vi "Process.vi"(8 "error in":errorcluster, 11 "Example Instrument UI":refnum<class "Instrument UI.LN2.lvclass">) -> (0 "error out":errorcluster, 3 "Example Instrument UI out":refnum<class "Instrument UI.LN2.lvclass">)   [LabVIEW 2019, in "Instrument UI.LN2.lvclass"]
doc: "---------------------------------------------------------------\nJKI State Machine Objects™\nhttp://jki.net/state-machine-objects/\nCopyright (C) 2005-2015, JKI <info@jki.net>\nALL RIGHTS RESERVEDJKI State Machine Objects (SMO) 1.0.0.5\nJKI - JKI\nCopyright (c) 2016, JKI"
uses:
  Instrument UI.LN2.lvclass
  C:/Program Files (x86)/National Instruments/LabVIEW 2019/vi.lib/JKI/JKI SMO/SMO/SMO.lvclass
  C:/Program Files (x86)/National Instruments/LabVIEW 2019/user.lib/LevyLab/Instrument Framework/SMOs/Instrument UI/Instrument UI.lvclass
  C:/Program Files (x86)/National Instruments/LabVIEW 2019/vi.lib/JKI/JKI SMO/SMO.UI/SMO.UI.lvclass
  Instrument.LN2/Typedefs/Instrument.LN2.getAll--Cluster.ctl
  Instrument.LN2/Instrument.LN2.lvclass
  C:/Program Files (x86)/National Instruments/LabVIEW 2019/user.lib/LevyLab/Instrument Framework/SMOs/Instrument/Instrument.lvclass
  Instrument UI.LN2.UI--Cluster.ctl
  Instrument.LN2/Typedefs/Instrument.LN2.Configuration--Cluster.ctl
  <userlib>/LevyLab/Instrument Framework/SMOs/Configuration/Configuration.lvclass
  <userlib>/LevyLab/Instrument Framework/SMOs/Instrument UI/Instrument UI.lvclass/Instrument UI.ctl
  <vilib>/JKI/JKI SMO/SMO/SMO.lvclass/SMO.ctl
  <userlib>/LevyLab/Instrument Framework/SMOs/Configuration/Configuration.lvclass/Configuration.ctl
  <userlib>/LevyLab/Instrument Framework/SMOs/Instrument/Instrument.lvclass/Instrument.ctl
  570207f0-e501-44f0-9618-964b5be4b2e0.vi
  064e3a37-d4cf-416d-9c97-81a00de9d50c.vi
  3ac88aea-1a9b-4987-becd-cafda593f7dd.vi
  <vilib>/JKI/JKI SMO/SMO/Private/ReftoDVR--SMO.vi
  570207f0-e501-44f0-9618-964b5be4b2e0.vi/caf046b2-5564-4fc5-9988-a6deaa861af8.vi
  064e3a37-d4cf-416d-9c97-81a00de9d50c.vi/e94c7b98-807a-4028-bf59-40b0245fb82b.vi
  3ac88aea-1a9b-4987-becd-cafda593f7dd.vi/dcf467b4-f1e1-4b46-b912-9ef69395c1ef.vi
  <userlib>/LevyLab/Instrument Framework/SMOs/Instrument/API/Send and Receive.vi
  3ac88aea-1a9b-4987-becd-cafda593f7dd.vi/87cdbc2a-7ef5-4e78-ae8f-77a685c984f9.vi
  <userlib>/LevyLab/Instrument Framework/SMOs/Instrument/Private/Get Client Type.vi
  570207f0-e501-44f0-9618-964b5be4b2e0.vi/caf046b2-5564-4fc5-9988-a6deaa861af8.vi/24e8312f-bad0-4d20-b7ce-0262f896184e.vi
  570207f0-e501-44f0-9618-964b5be4b2e0.vi/caf046b2-5564-4fc5-9988-a6deaa861af8.vi/d2585e3b-91c6-4f37-8627-ecef36f0e358.vi
  064e3a37-d4cf-416d-9c97-81a00de9d50c.vi/e94c7b98-807a-4028-bf59-40b0245fb82b.vi/ea1ec72b-e595-4509-9838-8d04b7e19cf0.vi
  064e3a37-d4cf-416d-9c97-81a00de9d50c.vi/e94c7b98-807a-4028-bf59-40b0245fb82b.vi/ca603f86-ca35-4c9c-a60a-82e1144c324f.vi
  3ac88aea-1a9b-4987-becd-cafda593f7dd.vi/dcf467b4-f1e1-4b46-b912-9ef69395c1ef.vi/e6b65ff1-2ffe-43b7-9398-b93f85180f35.vi
  3ac88aea-1a9b-4987-becd-cafda593f7dd.vi/dcf467b4-f1e1-4b46-b912-9ef69395c1ef.vi/e65e6366-964f-4408-b43e-2679365e4603.vi
  3ac88aea-1a9b-4987-becd-cafda593f7dd.vi/87cdbc2a-7ef5-4e78-ae8f-77a685c984f9.vi/814d43a9-fe47-4414-b08c-5bce024554fc.vi
  3ac88aea-1a9b-4987-becd-cafda593f7dd.vi/87cdbc2a-7ef5-4e78-ae8f-77a685c984f9.vi/5fb6644c-4c1d-4bef-b719-91b55b7f173d.vi
  570207f0-e501-44f0-9618-964b5be4b2e0.vi/caf046b2-5564-4fc5-9988-a6deaa861af8.vi/24e8312f-bad0-4d20-b7ce-0262f896184e.vi/2d73064b-1846-4431-93a5-eb87277d2863.vi
  570207f0-e501-44f0-9618-964b5be4b2e0.vi/caf046b2-5564-4fc5-9988-a6deaa861af8.vi/24e8312f-bad0-4d20-b7ce-0262f896184e.vi/96192298-3fd9-4fdc-9165-8347bdbd3bd8.vi
  570207f0-e501-44f0-9618-964b5be4b2e0.vi/caf046b2-5564-4fc5-9988-a6deaa861af8.vi/d2585e3b-91c6-4f37-8627-ecef36f0e358.vi/2d53ec29-cb0a-4d87-bfb8-ac7d7758049e.vi
  570207f0-e501-44f0-9618-964b5be4b2e0.vi/caf046b2-5564-4fc5-9988-a6deaa861af8.vi/d2585e3b-91c6-4f37-8627-ecef36f0e358.vi/68b74ad3-6d49-41d6-a3f9-22d3dbfe5c7c.vi
  064e3a37-d4cf-416d-9c97-81a00de9d50c.vi/e94c7b98-807a-4028-bf59-40b0245fb82b.vi/ea1ec72b-e595-4509-9838-8d04b7e19cf0.vi/e084a756-656f-4cb3-b7ce-ba8ae6e9a3ed.vi
  064e3a37-d4cf-416d-9c97-81a00de9d50c.vi/e94c7b98-807a-4028-bf59-40b0245fb82b.vi/ea1ec72b-e595-4509-9838-8d04b7e19cf0.vi/8cc34da9-8e4d-45ae-b786-ca14aa9f429e.vi
  064e3a37-d4cf-416d-9c97-81a00de9d50c.vi/e94c7b98-807a-4028-bf59-40b0245fb82b.vi/ca603f86-ca35-4c9c-a60a-82e1144c324f.vi/edcbe473-f127-4b1e-aea6-5a49f1961ddd.vi
  064e3a37-d4cf-416d-9c97-81a00de9d50c.vi/e94c7b98-807a-4028-bf59-40b0245fb82b.vi/ca603f86-ca35-4c9c-a60a-82e1144c324f.vi/9a19d119-1846-4deb-b3ac-a3b5d50ecf35.vi
  3ac88aea-1a9b-4987-becd-cafda593f7dd.vi/87cdbc2a-7ef5-4e78-ae8f-77a685c984f9.vi/814d43a9-fe47-4414-b08c-5bce024554fc.vi/aa77fdb9-b955-481b-814e-f9653af26bf2.vi
  3ac88aea-1a9b-4987-becd-cafda593f7dd.vi/87cdbc2a-7ef5-4e78-ae8f-77a685c984f9.vi/814d43a9-fe47-4414-b08c-5bce024554fc.vi/eac67a51-df62-4b9b-b6ca-6b8735c11697.vi
  570207f0-e501-44f0-9618-964b5be4b2e0.vi/caf046b2-5564-4fc5-9988-a6deaa861af8.vi/d2585e3b-91c6-4f37-8627-ecef36f0e358.vi/2d53ec29-cb0a-4d87-bfb8-ac7d7758049e.vi/17da7eab-c41b-4105-b235-6a3dd260d5b4.vi
  570207f0-e501-44f0-9618-964b5be4b2e0.vi/caf046b2-5564-4fc5-9988-a6deaa861af8.vi/d2585e3b-91c6-4f37-8627-ecef36f0e358.vi/2d53ec29-cb0a-4d87-bfb8-ac7d7758049e.vi/4a0639b9-f07b-4c56-94f4-68eb7f7105d7.vi
  064e3a37-d4cf-416d-9c97-81a00de9d50c.vi/e94c7b98-807a-4028-bf59-40b0245fb82b.vi/ca603f86-ca35-4c9c-a60a-82e1144c324f.vi/edcbe473-f127-4b1e-aea6-5a49f1961ddd.vi/a9985013-86db-4bf4-88b6-4de333bcf681.vi
  064e3a37-d4cf-416d-9c97-81a00de9d50c.vi/e94c7b98-807a-4028-bf59-40b0245fb82b.vi/ca603f86-ca35-4c9c-a60a-82e1144c324f.vi/edcbe473-f127-4b1e-aea6-5a49f1961ddd.vi/f3a922f7-f720-4162-b0c1-e020b75b8308.vi
  <userlib>/LevyLab/Instrument Framework/SMOs/Instrument/Private/Get RC Connection Status.vi
  <userlib>/LevyLab/Instrument Framework/SMOs/Instrument/API/Enum to String.vi
  <userlib>/LevyLab/Instrument Framework/SMOs/RemoteControl/API/Send and Receive.vi
  <vilib>/Utility/Data Type/Get Type Information.vi
  <vilib>/JDP Science/JSONtext/JSON text to Variant.vi
  <vilib>/JDP Science/JSONtext/Variant to JSON Text.vi
  <vilib>/National Instruments/GUID Generator/Guid Generator.vi
  <userlib>/LevyLab/Instrument Framework/SMOs/Instrument/Private/Instrument.MessageFromProcess.EventStructure.vi
  <userlib>/LevyLab/Instrument Framework/SMOs/Instrument/Instrument.lvclass
  <vilib>/JDP Science/JSONtext/LVClass Serializer/JSONtext LVClass Serializer.lvclass
  <userlib>/LevyLab/Instrument Framework/SMOs/Instrument UI/Instrument UI.lvclass
  <vilib>/JKI/JKI SMO/SMO/SMO.lvclass
  <vilib>/JKI/JKI SMO/SMO.UI/SMO.UI.lvclass
panel:
  out "Net weight":dbl
  in  "set empty weight":bool
  out "Level (%)":dbl(slide) scale=0.0..100.0
  out "Numeric":u32
  in  "set full weight":bool
  in  "STOP":bool
  # "SMO UI Template"
  # "For instructions on how to use the JKI State Machine Objects, examples and video tutorials, visit:\nhttp://jki.net/state-machine-objects/\n\nJKI State Machine Objects™\nhttp://jki.net/state-machine-objects/\nCopyright (C) 2005-2015, JKI <info@jki.net>\nALL RIGHTS RESERVED"
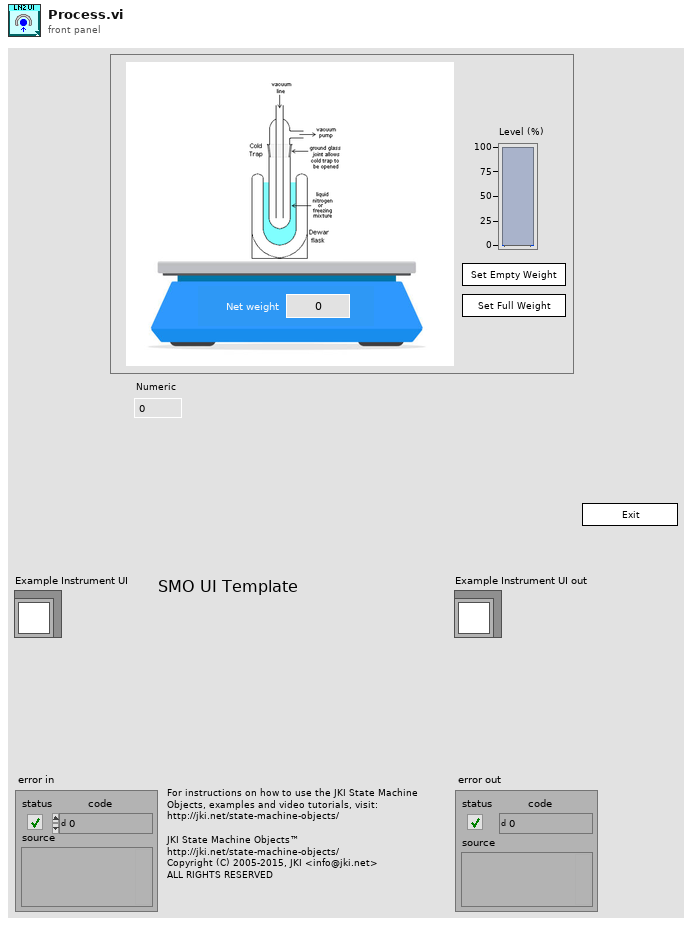
[diagram p1: front panel]
types:
  T1 = enum32{"invalid app kind", "Development System", "Run Time System", "Student Edition", "Embedded LabVIEW", "Evaluation", "Custom"}
  T2 = enum32{"Invalid", "Standard", "Closed", "Hidden", "Minimized", "Maximized"}
  T3 = typedef "Instrument.LN2.lvclass/Instrument.LN2.Configuration--Cluster.ctl" = cluster{"Example Setting 1":dbl, "Example Setting 2":dbl, "Example Setting 3":string}
  T4 = typedef "Instrument.LN2.lvclass/Instrument.LN2.getAll--Cluster.ctl" = cluster{"Net Weight(lbs)":dbl, "Gross Weight(lbs) ":dbl, "Tare Weight(lbs) ":dbl, "Empty":dbl}
  T5 = typedef "Instrument UI.LN2.lvclass/Instrument UI.LN2.UI--Cluster.ctl" = cluster{"empty weight":dbl, "full weight":dbl}
  T6 = cluster{"Core":cluster{"Current VI Reference":refnum<vi>, "Close Panel on Exit?":bool, "error":errorcluster}, "Instrument UI":refnum<class "Instrument UI.LN2.lvclass">, "Instrument":refnum<class "Instrument.LN2.lvclass">, "Configuration":refnum<class "Configuration.lvclass">, "Config Cluster":T3, "getAll":T4, "UI Cluster":T5}
  T7 = cluster{"Current VI Reference":refnum<vi>, "Close Panel on Exit?":bool, "error":errorcluster}
  T8 = typedef "SMO.lvclass/Protected Events.ctl" = cluster{"StopProcesses":refnum<user-event>, "AbortProcesses":refnum<user-event>, "Config Changed":refnum<user-event>, "Dependency":refnum<user-event>}
  T9 = typedef "Instrument.lvclass/PublicEvents--Cluster.ctl" = cluster{"MessageFromProcess":refnum<user-event>}
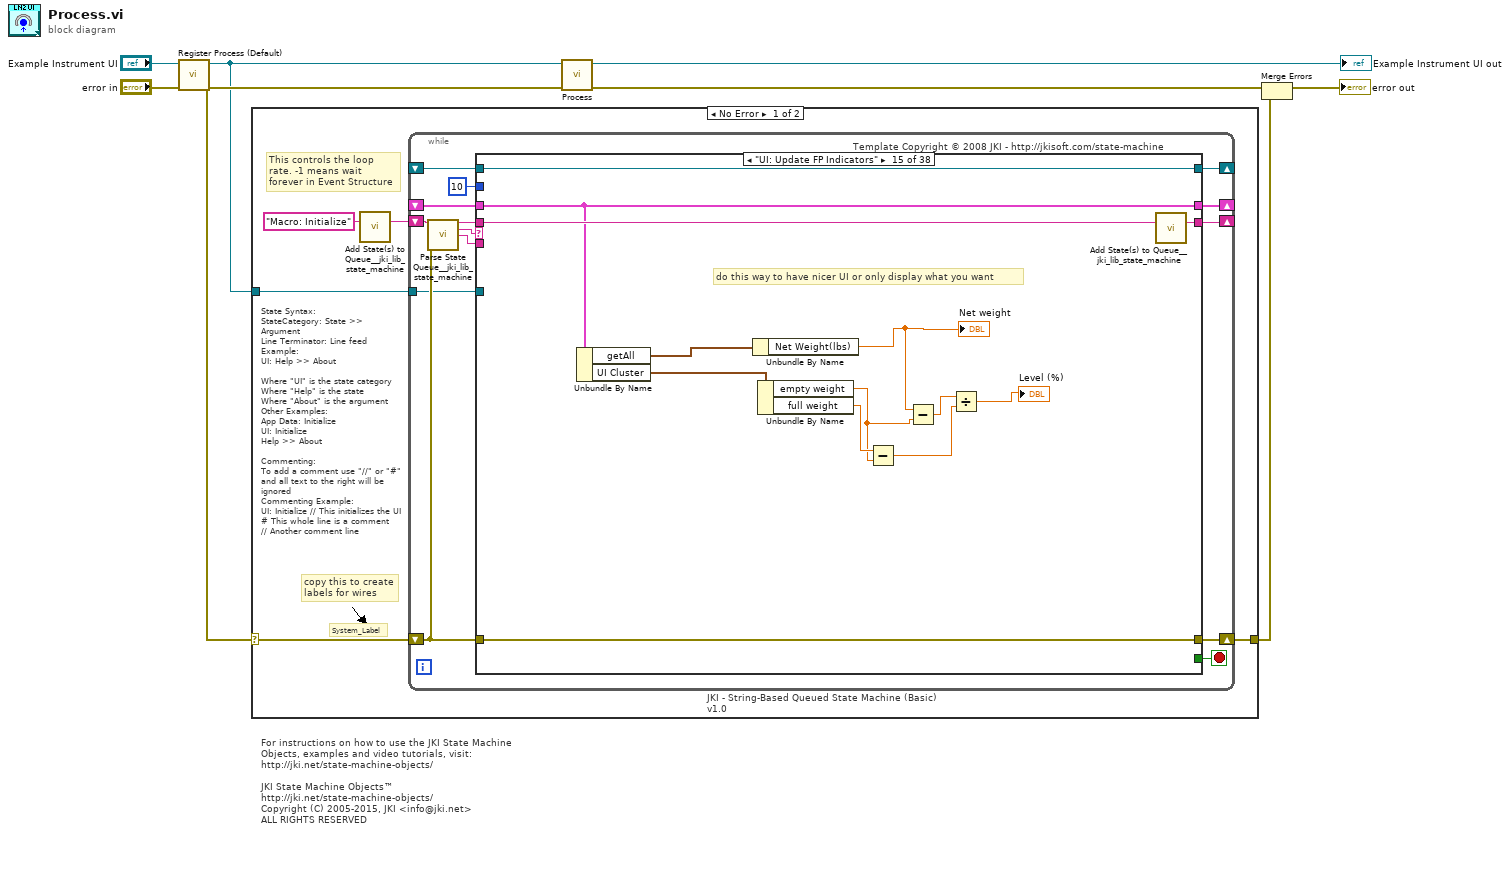
[diagram p0: block diagram]
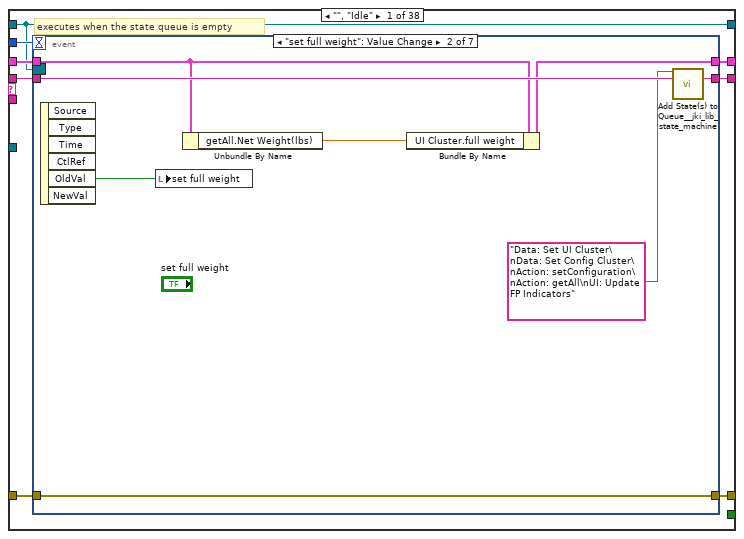
[diagram p2: hidden frame]
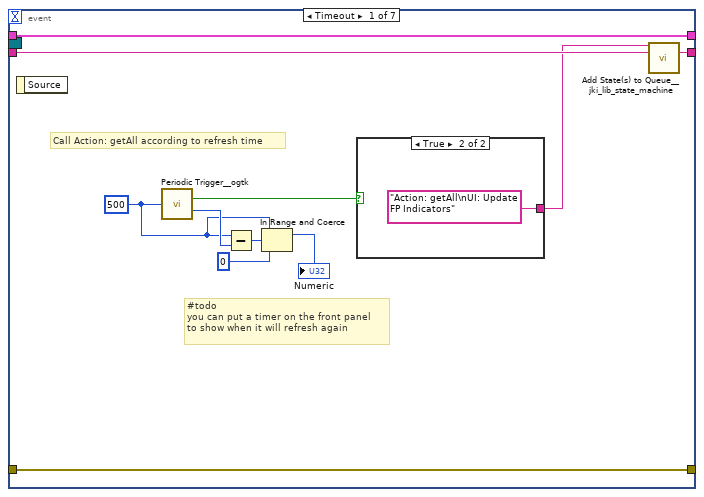
[diagram p3: hidden frame]
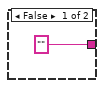
[diagram p4: hidden frame]
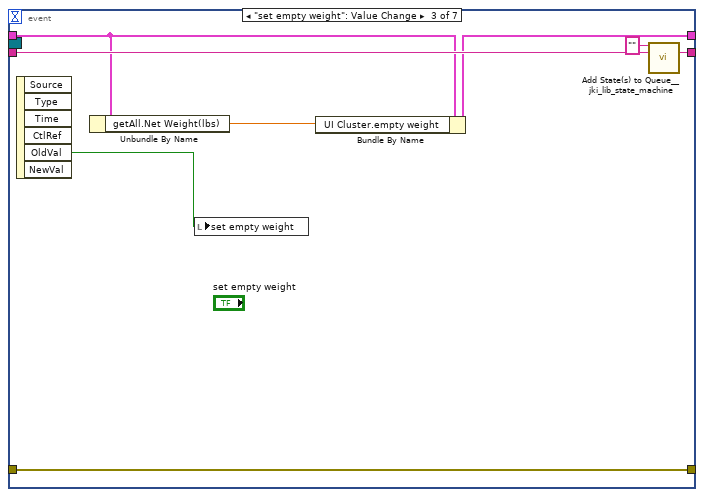
[diagram p5: hidden frame]
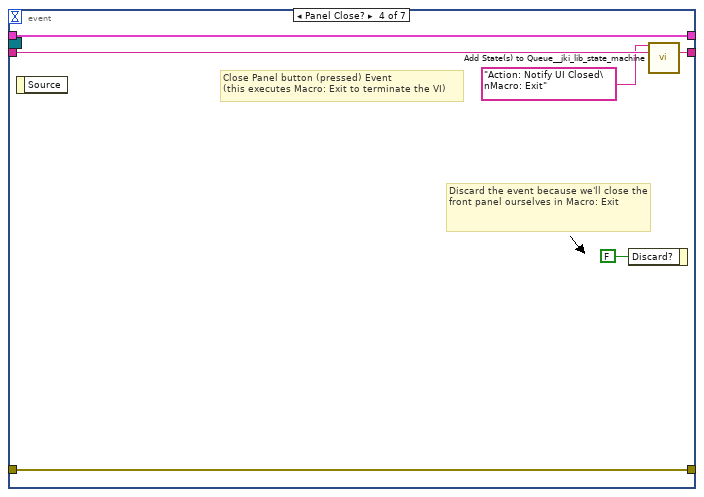
[diagram p6: hidden frame]
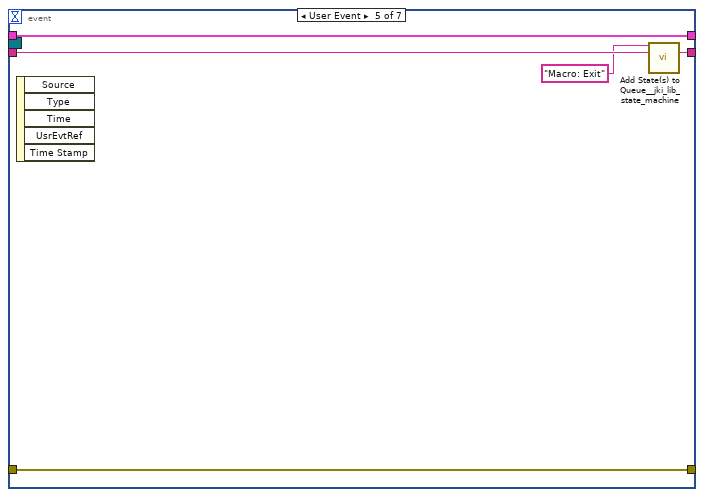
[diagram p7: hidden frame]
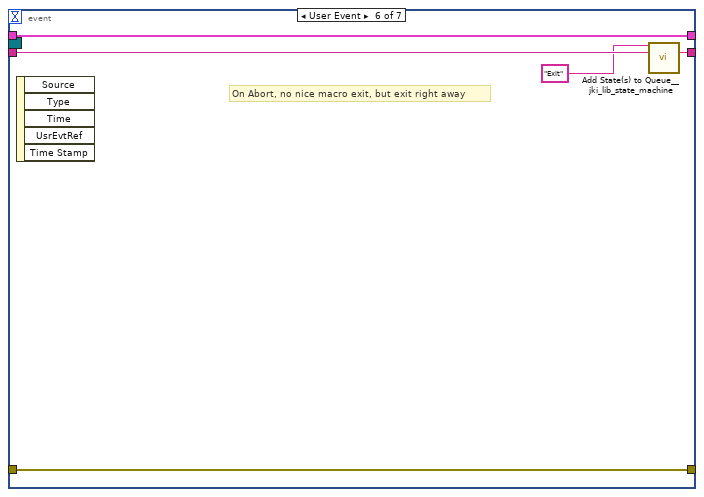
[diagram p8: hidden frame]
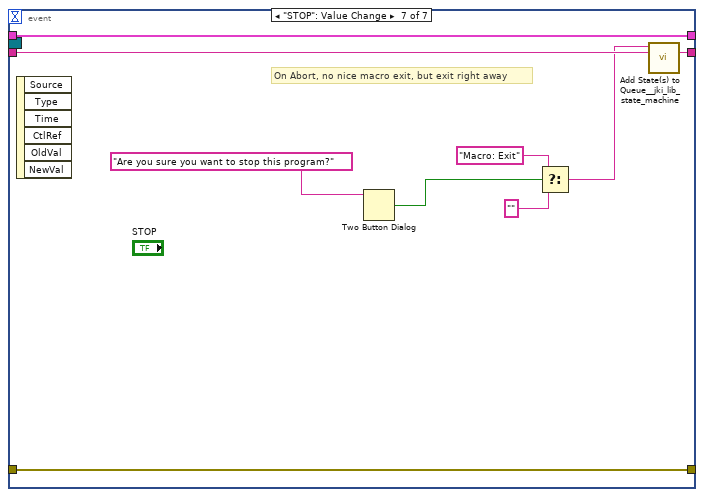
[diagram p9: hidden frame]
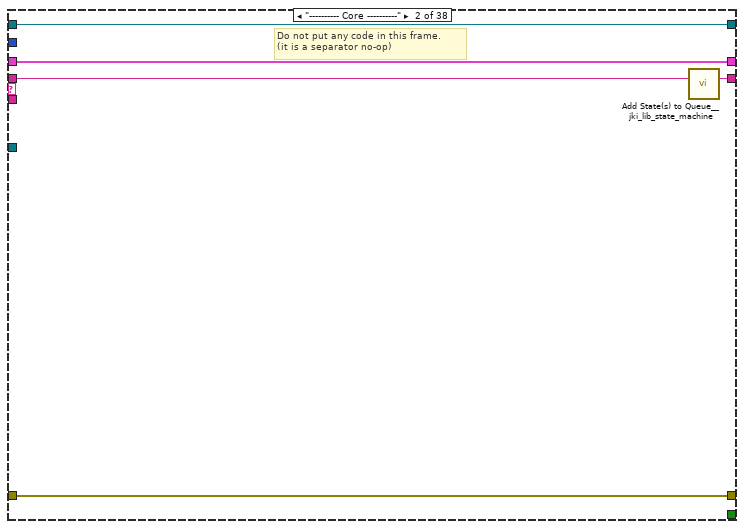
[diagram p10: hidden frame]
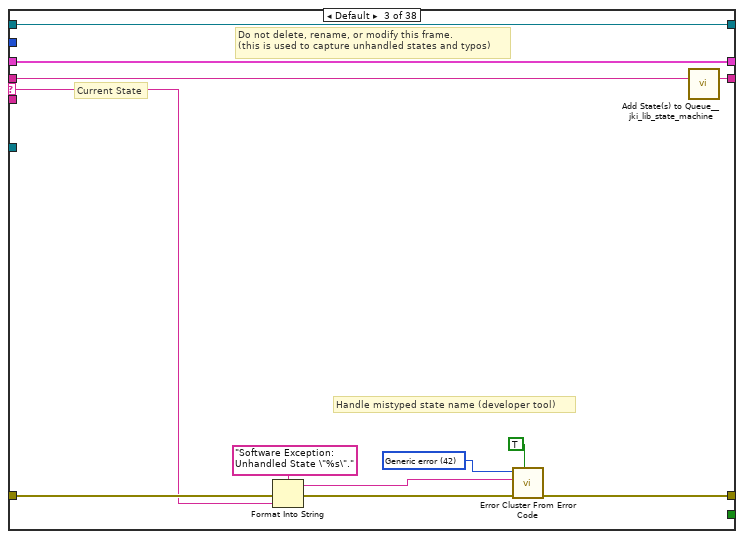
[diagram p11: hidden frame]
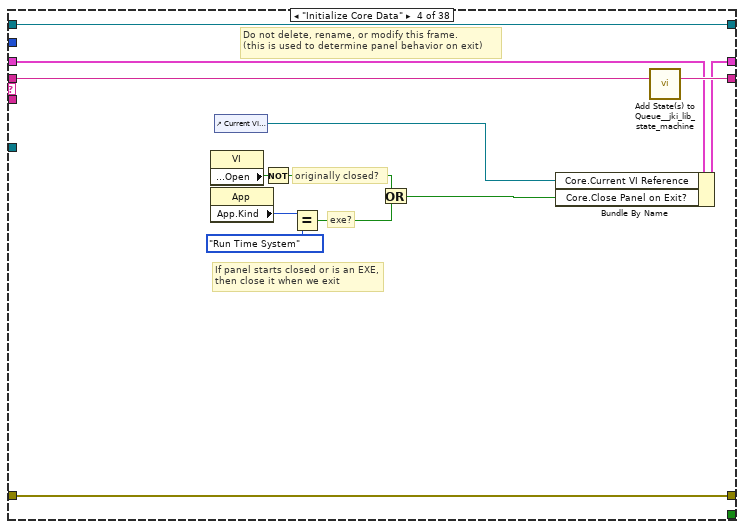
[diagram p12: hidden frame]
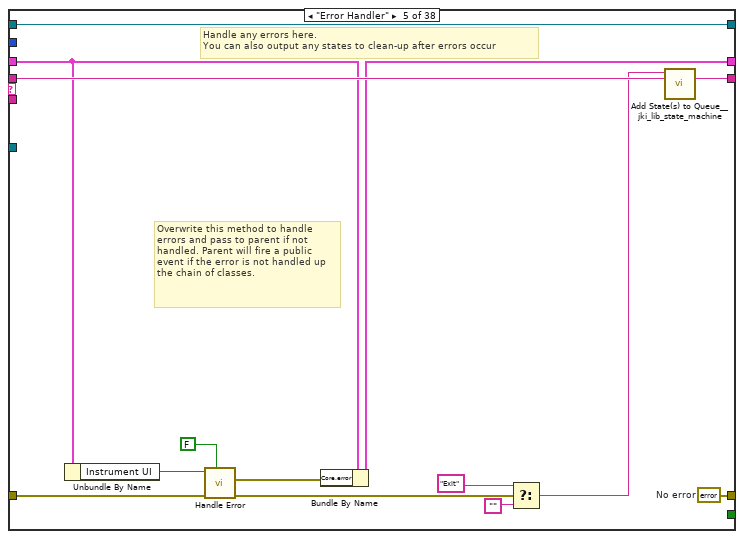
[diagram p13: hidden frame]
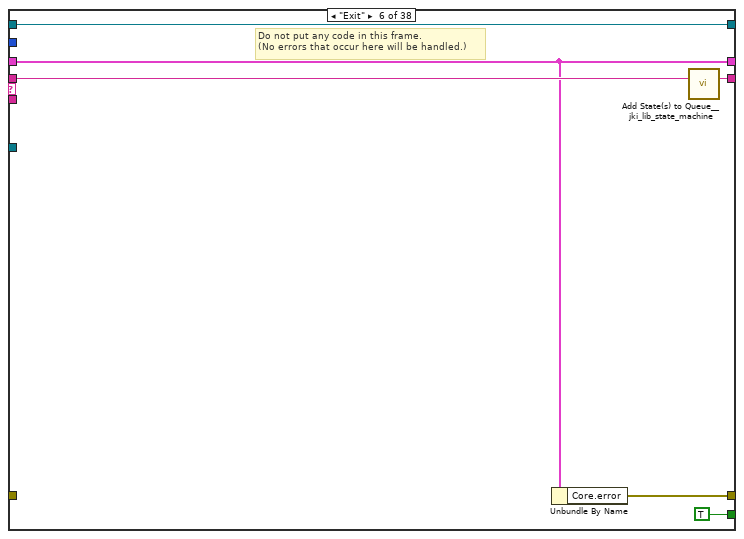
[diagram p14: hidden frame]
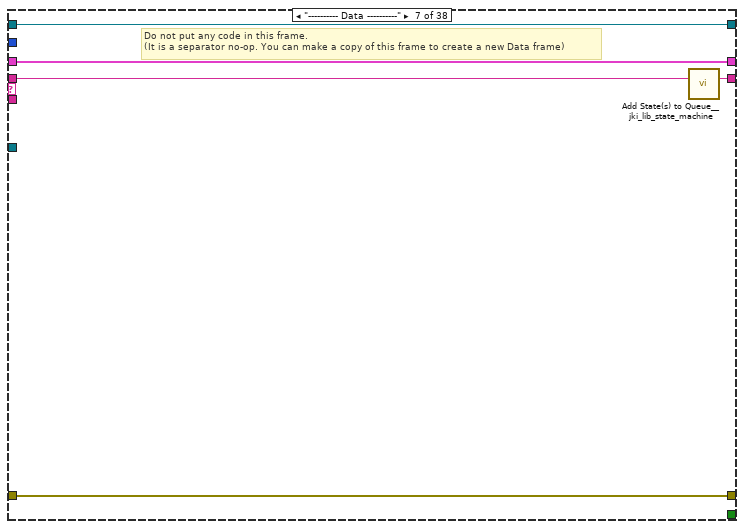
[diagram p15: hidden frame]
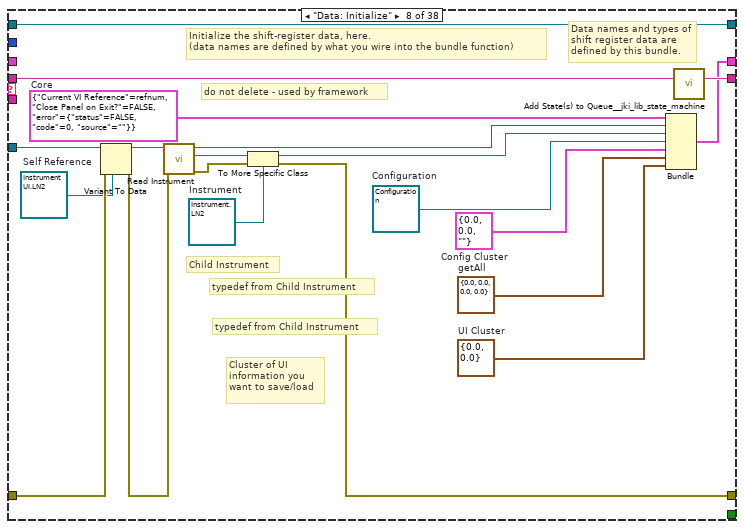
[diagram p16: hidden frame]
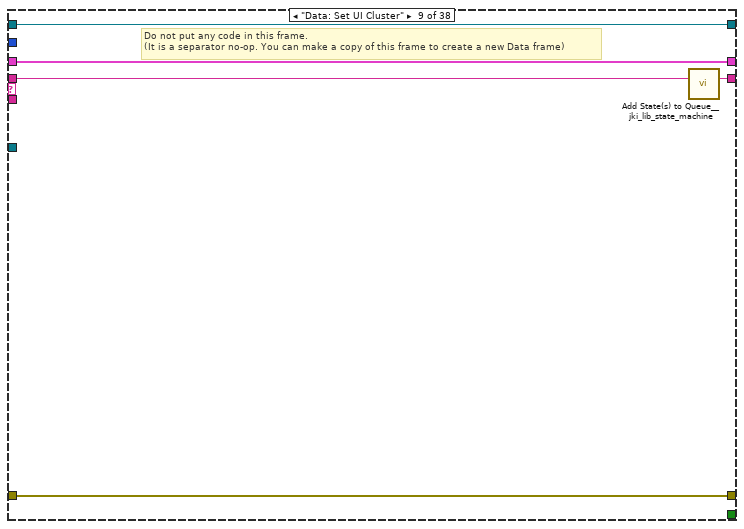
[diagram p17: hidden frame]
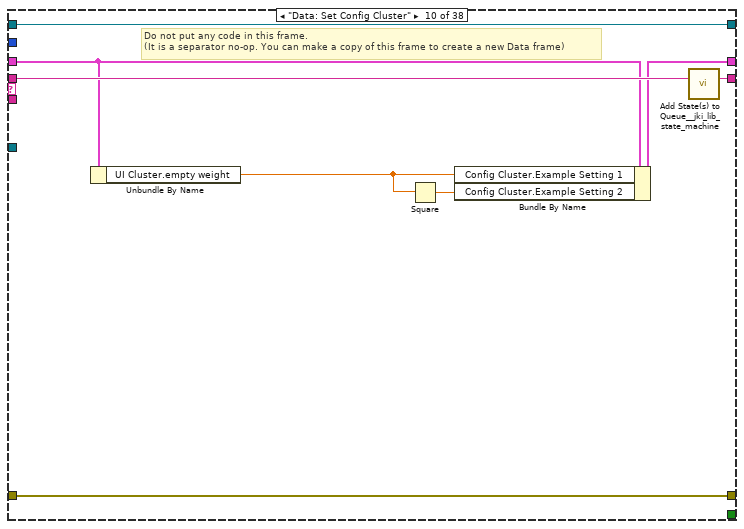
[diagram p18: hidden frame]
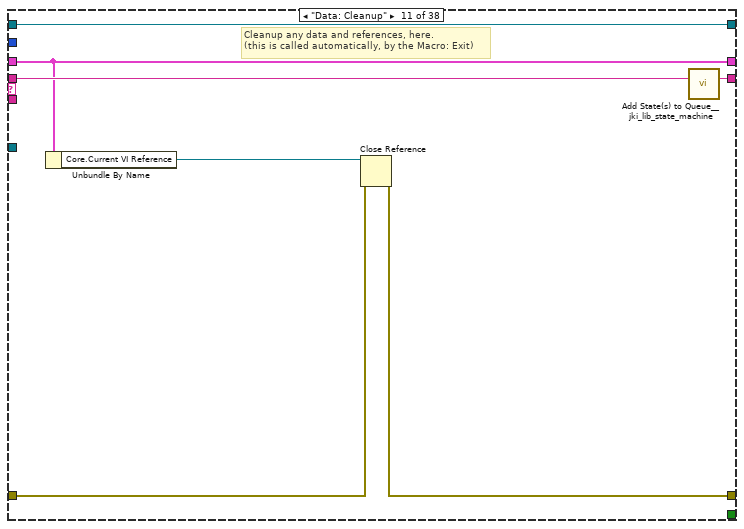
[diagram p19: hidden frame]
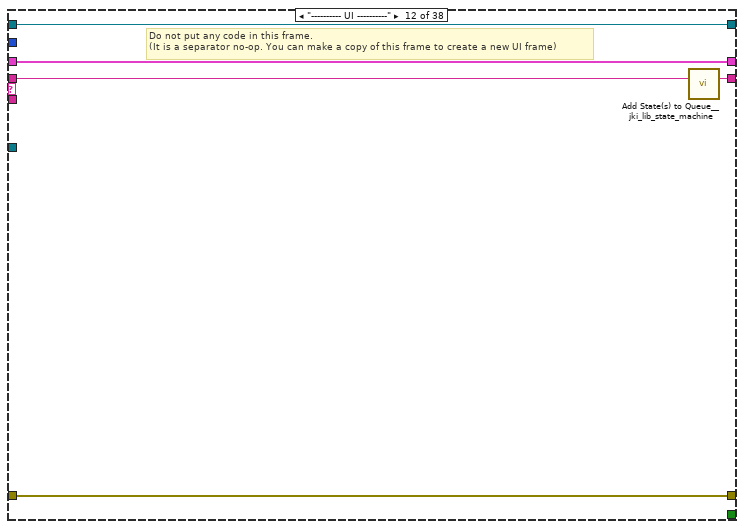
[diagram p20: hidden frame]
diagram:
  # "For instructions on how to use the JKI State Machine Objects, examples and video tutorials, visit:\nhttp://jki.net/state-machine-objects/\n\nJKI State Machine Objects™\nhttp://jki.net/state-machine-objects/\nCopyright (C) 2005-2015, JKI <info@jki.net>\nALL RIGHTS RESERVED"
  n1 = call <vilib>:"Register Process (Default).vi"("error in (no error)"="error in", "SMO"="Example Instrument UI") -> ("error out"=w5:errorcluster, "SelfRef"=w4:refnum<class "Instrument UI.LN2.lvclass">)  [unwired: 8 in]
  n2 = case shown="No Error" w5 {
    selector: w5 -> [w10 w450]
    tunnel: w4 -> [w11 _]
    tunnel: [w9 w450] -> w1
    frame No Error {
      # "State Syntax:\nStateCategory: State >> Argument\nLine Terminator: Line feed\nExample:\nUI: Help >> About\n\nWhere \"UI\" is the state category\nWhere \"Help\" is the state\nWhere \"About\" is the argument\nOther Examples:\nApp Data: Initialize\nUI: Initialize\nHelp >> About\n\nCommenting:\nTo add a comment use \"//\" or \"#\" and all text to the right will be ignored\nCommenting Example:\nUI: Initialize // This initializes the UI\n# This whole line is a comment\n// Another comment line"
      # "copy this to create labels for wires"
      # "This controls the loop rate. -1 means wait forever in Event Structure"
      # "System_Label"
      n3 = call <vilib>:"Add State(s) to Queue__jki_lib_state_machine.vi"("State(s) in (\"\")"="Macro: Initialize") -> ("States Out"=w13:string)  [unwired: 14 in]
      n4 = while "JKI - String-Based Queued State Machine (Basic) v1.0" {
        shift-right: [w20] -> _
        shift-left: _ -> [w19]
        shift-right: [w23] -> w9
        shift-left: w10 -> [w17]
        shift-right: [w22] -> _
        shift-left: w13 -> [w24]
        tunnel: w11 -> [w16]
        shift-right: [w15] -> _
        shift-left: _ -> [w14]
        stop <- w21 stop-if-true
        # "Template Copyright © 2008 JKI - http://jkisoft.com/state-machine"
        n5 = call <vilib>:"Parse State Queue__jki_lib_state_machine.vi"("State Queue"=w24, "Error In (no error)"=w17) -> ("Remaining States"=w26:string, "Current State"=w27:string, "Arguments"=w25:string)  [unwired: 11 in]
        n6 = case shown="\"UI: Update FP Indicators\"" w27 {
          selector: w27 -> [_ _ w96 _ _ _ _ _ _ _ _ _ _ _ _ _ _ _ _ _ _ _ _ _ _ _ _ _ _ _ _ _ _ _ _ _ _ _]
          tunnel: w26 -> [w35 w94 w100 w119 w133 w139 w144 w164 w169 w177 w184 w189 w196 w203 w216 w223 w239 w271 w280 w286 w292 w307 w312 w323 w330 w335 w348 w354 w359 w374 w382 w394 w401 w408 w420 w431 w440 w449]
          tunnel: w25 -> [_ _ _ _ _ _ _ _ _ _ _ _ _ _ _ w217 w233 _ _ _ _ _ _ _ _ _ _ _ _ _ _ _ _ _ _ _ _ _]
          tunnel: w19 -> [w33 w91 w98 w110 w122 w135 w141 _ w165 w173 w178 w186 w194 w199 w211 w221 w235 w268 w276 w283 w289 w294 w309 w320 w325 w332 w346 w352 w356 w367 w379 w385 w397 w402 w415 w423 w436 w445]
          tunnel: [w32 w92 w102 w116 w124 w134 w142 w146 w167 w175 w180 w187 w191 w201 w212 w218 w236 w269 w278 w284 w290 w305 w310 w314 w326 w333 w341 w349 w357 w361 w377 w386 w398 w403 w410 w428 w437 w446] -> w23
          tunnel: w17 -> [w31 w92 w101 w116 w129 _ w142 w161 w167 w175 w181 w187 w192 w201 w212 w219 w237 w269 w278 w284 w290 w305 w310 w315 w327 w333 w343 w350 w357 w369 w375 w387 w398 w404 w411 w424 w437 w446]
          tunnel: [w34 w93 w99 w118 w132 w138 w143 w163 w168 w176 w183 w188 w195 w202 w215 w222 w238 w270 w279 w285 w291 w306 w311 w322 w329 w334 w347 w353 w358 w373 w381 w393 w400 w407 w419 w430 w439 w448] -> w22
          tunnel: [_ _ _ _ _ TRUE _ _ _ _ _ _ _ _ _ _ _ _ _ _ _ _ _ _ _ _ _ _ _ _ _ _ _ _ _ _ _ _] -> w21
          tunnel: [w30 w91 w98 w117 w121 w135 w141 w162 w165 w172 w178 w186 w194 w199 w211 w221 w235 w268 w276 w283 w289 w294 w309 w320 w325 w332 w346 w352 w356 w371 w379 w383 w396 w402 w416 w425 w435 w444] -> w20
          tunnel: 10 ("Timeout") -> [w29 _ _ _ _ _ _ _ _ _ _ _ _ _ _ _ _ _ _ _ _ _ _ _ _ _ _ _ _ _ _ _ _ _ _ _ _ _]
          tunnel: w16 -> [_ _ _ _ _ _ _ w159 _ _ _ _ _ _ _ _ _ _ _ _ _ _ _ _ _ _ _ _ _ _ _ _ _ _ _ _ _ _]
          tunnel: [w28 w90 w95 w107 w131 w136 w140 w158 w166 w174 w179 w185 w193 w200 w214 w220 w232 w267 w277 w282 w288 w299 w308 w321 w328 w331 w345 w351 w355 w372 w380 w392 w399 w406 w418 w429 w438 w447] -> w15
          tunnel: w14 -> [w28 w90 w95 w107 w131 w136 w140 w158 w166 w174 w179 w185 w193 w200 w214 w220 w232 w267 w277 w282 w288 w299 w308 w321 w328 w331 _ w351 w355 w372 w380 w392 w399 w406 w418 w429 w438 w447]
          frame "", "Idle" {
            # "executes when the state queue is empty"
            n7 = event shown="[1] \"set full weight\": Value Change" {
              selector: w28 -> [_ _ _ _ _ _ _]
              dyn-events: _ -> [_ _ _ _ _ _ _]
              timeout: w29 -> [_ _ _ _ _ _ _]
              tunnel: w35 -> [w46 w56 w64 w70 w75 w80 w89]
              tunnel: [w45 w55 w63 w69 w74 w79 w88] -> w34
              tunnel: w33 -> [w43 w51 w59 w66 w72 w77 w86]
              tunnel: [w44 w54 w62 w65 w73 w78 w87] -> w32
              tunnel: w31 -> [w44 w54 w62 w65 w73 w78 w87]
              tunnel: [w43 w52 w61 w66 w72 w77 w86] -> w30
              event Timeout {
                w37 = u32 500 ("time (ms)")
                # "#todo\nyou can put a timer on the front panel\nto show when it will refresh again"
                # "Call Action: getAll according to refresh time"
                n8 = event-data() -> ()  [unwired: 1 in, 1 out]
                n9 = call <userlib>:"Periodic Trigger__ogtk.vi"("time (ms)"=w37) -> ("Triggered"=w41:bool, "timer value"=w40:u32)  [unwired: 12 in, 1 out]
                n10 = Subtract(x=w37, y=w40) -> (x-y=w39:u32)
                n11 = In Range and Coerce(upper limit=w37, x=w39, lower limit=u32 0) -> (coerced(x)=→"Numeric":u32)  [unwired: 1 out]
                n12 = case shown="True" w41 {
                  tunnel: ["" ("State(s) in Front (\"\")") "Action: getAll\nUI: Update FP Indicators" ("State(s) in Front (\"\")")] -> w42
                  frame False {
                  }
                  frame True {
                  }
                }
                n13 = call <vilib>:"Add State(s) to Queue__jki_lib_state_machine.vi"("State(s) in Front (\"\")"=w42, "State(s) in (\"\")"=w46) -> ("States Out"=w45:string)  [unwired: 13 in]
              }
              event "set full weight": Value Change {
                n14 = event-data() -> ("OldVal"=w49:bool)  [unwired: 1 in, 5 out]
                n15 = local write "set full weight"(w49) -> ()
                n16 = Unbundle By Name(w51) -> ("getAll.Net Weight(lbs)"=w50:dbl)
                n17 = Bundle By Name(cluster=w51, "UI Cluster.full weight"=w50) -> (w52:T6)
                n18 = call <vilib>:"Add State(s) to Queue__jki_lib_state_machine.vi"("State(s) in Front (\"\")"="Data: Set UI Cluster\nData: Set Config Cluster\nAction: setConfiguration\nAction: getAll\nUI: Update FP Indicators" ("State(s) in Front (\"\")"), "State(s) in (\"\")"=w56) -> ("States Out"=w55:string)  [unwired: 13 in]
              }
              event "set empty weight": Value Change {
                n19 = event-data() -> ("OldVal"=w57:bool)  [unwired: 1 in, 5 out]
                n20 = Unbundle By Name(w59) -> ("getAll.Net Weight(lbs)"=w58:dbl)
                n21 = local write "set empty weight"(w57) -> ()
                n22 = Bundle By Name(cluster=w59, "UI Cluster.empty weight"=w58) -> (w61:T6)
                n23 = call <vilib>:"Add State(s) to Queue__jki_lib_state_machine.vi"("State(s) in Front (\"\")"="" ("State(s) in Front (\"\")"), "State(s) in (\"\")"=w64) -> ("States Out"=w63:string)  [unwired: 13 in]
              }
              event Panel Close? {
                # "Discard the event because we'll close the front panel ourselves in Macro: Exit"
                # "Close Panel button (pressed) Event\n(this executes Macro: Exit to terminate the VI)"
                n24 = event-data() -> ()  [unwired: 1 in, 1 out]
                n25 = event-data("Discard?"=FALSE) -> ()  [unwired: 1 in, 1 out]
                n26 = call <vilib>:"Add State(s) to Queue__jki_lib_state_machine.vi"("State(s) in Front (\"\")"="Action: Notify UI Closed\nMacro: Exit", "State(s) in (\"\")"=w70) -> ("States Out"=w69:string)  [unwired: 13 in]
              }
              event User Event {
                n27 = event-data() -> ()  [unwired: 1 in, 5 out]
                n28 = call <vilib>:"Add State(s) to Queue__jki_lib_state_machine.vi"("State(s) in Front (\"\")"="Macro: Exit", "State(s) in (\"\")"=w75) -> ("States Out"=w74:string)  [unwired: 13 in]
              }
              event User Event {
                # "On Abort, no nice macro exit, but exit right away"
                n29 = event-data() -> ()  [unwired: 1 in, 5 out]
                n30 = call <vilib>:"Add State(s) to Queue__jki_lib_state_machine.vi"("State(s) in Front (\"\")"="Exit", "State(s) in (\"\")"=w80) -> ("States Out"=w79:string)  [unwired: 13 in]
              }
              event "STOP": Value Change {
                # "On Abort, no nice macro exit, but exit right away"
                n31 = event-data() -> ()  [unwired: 1 in, 6 out]
                n32 = Two Button Dialog(message="Are you sure you want to stop this program?") -> (T button?=w85:bool)  [unwired: 2 in]
                n33 = Select(t="Macro: Exit", s=w85, f="") -> (s? t:f=w81:string)
                n34 = call <vilib>:"Add State(s) to Queue__jki_lib_state_machine.vi"("State(s) in Front (\"\")"=w81, "State(s) in (\"\")"=w89) -> ("States Out"=w88:string)  [unwired: 13 in]
              }
            }
          }
          frame "---------- Core ----------" {
            # "Do not put any code in this frame.\n(it is a separator no-op)"
            n35 = call <vilib>:"Add State(s) to Queue__jki_lib_state_machine.vi"("State(s) in (\"\")"=w94) -> ("States Out"=w93:string)  [unwired: 14 in]
          }
          frame Default {
            w105 = 42 items=["No error", "Argument error", "Memory is full", "Out of zone", "End of file", "File already open", "Generic file I/O error", "File not found", "File permission error", "Disk is full", "Duplicate path", "Too many files open", "System feature not enabled", "Resource file not found", "Cannot add resource", "Resource not found", "Image not found", "Image memory error", "Pen does not exist", "Config type invalid", "Config token not found", "Config parse error", "Config memory error", "Bad external code format", "Bad external code offset", "External code not present", "Null window", "Destroy window error", "Null menu", "Print aborted", "Bad print record", "Print driver error", "Windows error during printing", "Memory error during printing", "Print dialog error", "Generic print error", "Invalid device refnum", "Device not found", "Device parameter error", "Device unit error", "Cannot open device", "Device call aborted", "Generic error", "Cancelled by user", "Object ID too low", "Object ID too high", "Object not in heap", "Unknown heap", "Unknown object (invalid DefProc)", "Unknown object (DefProc not in table)", "Message out of range", "Invalid (null) method", "Unknown message", "Manager call not supported", "Bad address", "Network operation in progress", "Network operation timed out", "Connection is busy", "Network attribute not supported", "Network error", "Address in use", "System out of memory", "Connection aborted", "Connection refused", "Not connected", "Already connected", "Connection closed", "Initialization error (interapplication manager)", "Bad occurrence", "Wait on unbound occurrence handler", "Occurrence queue overflow", "Datalog type conflict", "Unused", "Unrecognized type (interapplication manager)", "Memory corrupt", "Failed to make temporary DLL", "Old CIN version", "Drag socket not found", "Failed to load drop-object", "Failed to register OLE object", "Failed to release OLE object", "Format specifier type mismatch", "Unknown format specifier", "Too few format specifiers", "Too many format specifiers", "Scan failed", "Newer CIN version", "Error converting to variant", "Runtime menu error", "Password tampered", "Variant attribute not found", "Incompatible variant data type", "Event data is not available", "Event Store is not present", "Occurrence is not found", "Event Queue is not created", "Event info is not available", "Refnum passed is NULL", "Error retrieving Class GUID", "Error retrieving CoClass GUID", "Error retrieving TypeLib GUID.", "Bad built application magic bytes.", "Specific driver is different from the specific driver associated with the Logical Name.", "There is no session opened to the class driver.", "Max Error", "MAX - Error with config objects", "MAX - Error loading configuration", "MAX - Group not supported"]
            # "Current State"
            # "Do not delete, rename, or modify this frame.\n(this is used to capture unhandled states and typos)"
            # "Handle mistyped state name (developer tool)"
            n36 = Format Into String(format string="Software Exception: Unhandled State \"%s\"." ("message"), error in=w101, w96) -> (resulting string=w104:string, error out=w103:errorcluster)  [unwired: 1 in]
            n37 = call <vilib>:"Error Cluster From Error Code.vi"("show call chain? (False)"=TRUE, "error in (no error)"=w103, "error message (\"\")"=w104, "error code (0)"=w105) -> ("error out"=w102:errorcluster)  [unwired: 5 in]
            n38 = call <vilib>:"Add State(s) to Queue__jki_lib_state_machine.vi"("State(s) in (\"\")"=w100) -> ("States Out"=w99:string)  [unwired: 14 in]
          }
          frame "Initialize Core Data" {
            # "Do not delete, rename, or modify this frame.\n(this is used to determine panel behavior on exit)"
            # "originally closed?"
            # "exe?"
            # "If panel starts closed or is an EXE, then close it when we exit"
            n39 = property class="VI"() -> ("Front Panel.Open"=w115:bool)  [unwired: 2 in, 2 out]
            n40 = property class="App"() -> ("App.Kind"=w114:T1)  [unwired: 2 in, 2 out]
            n41 = control-ref of="Current VI Reference"() -> (w108:refnum<vi>)
            n42 = Not(x=w115) -> (.not. x?=w112:bool)
            n43 = Equal?(x=w114, y=T1."Run Time System" ("Application:Kind")) -> (x = y?=w111:bool)
            n44 = Or(x=w112, y=w111) -> (x .or. y?=w109:bool)
            n45 = Bundle By Name(cluster=w110, "Core.Current VI Reference"=w108, "Core.Close Panel on Exit?"=w109) -> (w117:T6)
            n46 = call <vilib>:"Add State(s) to Queue__jki_lib_state_machine.vi"("State(s) in (\"\")"=w119) -> ("States Out"=w118:string)  [unwired: 14 in]
          }
          frame "Error Handler" {
            w124 = errorcluster {"status"=FALSE, "code"=0, "source"=""}  # No error
            # "Overwrite this method to handle errors and pass to parent if not handled. Parent will fire a public event if the error is not handled up the chain of classes."
            # "Handle any errors here.\nYou can also output any states to clean-up after errors occur"
            n47 = Unbundle By Name(w122) -> ("Instrument UI"=w130:refnum<class "Instrument UI.LN2.lvclass">)
            n48 = call-dynamic "Handle Error.vi"("Stop on Unhandled Error (T)"=FALSE, "error in"=w129, "SMO"=w130) -> ("handling error"=w125:errorcluster, "Unhandled error"=w123:errorcluster)  [unwired: 6 in, 1 out]
            n49 = Bundle By Name(cluster=w122, "Core.error"=w123) -> (w121:T6)
            n50 = Select(t="Exit", s=w125, f="") -> (s? t:f=w126:string)
            n51 = call <vilib>:"Add State(s) to Queue__jki_lib_state_machine.vi"("State(s) in Front (\"\")"=w126, "State(s) in (\"\")"=w133) -> ("States Out"=w132:string)  [unwired: 13 in]
          }
          frame "Exit" {
            # "Do not put any code in this frame.\n(No errors that occur here will be handled.)"
            n52 = Unbundle By Name(w135) -> ("Core.error"=w134:errorcluster)
            n53 = call <vilib>:"Add State(s) to Queue__jki_lib_state_machine.vi"("State(s) in (\"\")"=w139) -> ("States Out"=w138:string)  [unwired: 14 in]
          }
          frame "---------- Data ----------" {
            # "Do not put any code in this frame.\n(It is a separator no-op. You can make a copy of this frame to create a new Data frame)"
            n54 = call <vilib>:"Add State(s) to Queue__jki_lib_state_machine.vi"("State(s) in (\"\")"=w144) -> ("States Out"=w143:string)  [unwired: 14 in]
          }
          frame "Data: Initialize" {
            w145 = refnum<class "Configuration.lvclass"> refnum  # Configuration
            w148 = T3 {"Example Setting 1"=0.0, "Example Setting 2"=0.0, "Example Setting 3"=""}  # Config Cluster
            w150 = T5 {"empty weight"=0.0, "full weight"=0.0}  # UI Cluster
            w152 = refnum<class "Instrument.LN2.lvclass"> refnum  # Instrument
            w156 = T4 {"Net Weight(lbs)"=0.0, "Gross Weight(lbs) "=0.0, "Tare Weight(lbs) "=0.0, "Empty"=0.0}  # getAll
            w157 = T7 {"Current VI Reference"=refnum, "Close Panel on Exit?"=FALSE, "error"={"status"=FALSE, "code"=0, "source"=""}}  # Core
            w160 = refnum<class "Instrument UI.LN2.lvclass"> refnum  # Self Reference
            # "typedef from Child Instrument"
            # "Cluster of UI\ninformation you\nwant to save/load"
            # "Child Instrument"
            # "typedef from Child Instrument"
            # "do not delete - used by framework"
            # "Data names and types of shift register data are defined by this bundle."
            # "Initialize the shift-register data, here.\n(data names are defined by what you wire into the bundle function)"
            n55 = Variant To Data(error in=w161, type=w160, Variant=w159) -> (data=w154:refnum<class "Instrument UI.LN2.lvclass">, error out=w155:errorcluster)
            n56 = call <userlib>:"Read Instrument.vi"("error in (no error)"=w155, "Instrument UI in"=w154) -> ("error out"=w149:errorcluster, "Instrument"=w151:refnum<class "Instrument.lvclass">, "Instrument UI"=w153:refnum<class "Instrument UI.LN2.lvclass">)  [unwired: 7 in]
            n57 = To More Specific Class(target class=w152, reference=w151, error in=w149) -> (specific class reference=w147:refnum<class "Instrument.LN2.lvclass">, error out=w146:errorcluster)
            n58 = Bundle("Core"=w157, "Instrument UI"=w153, "Instrument"=w147, "Configuration"=w145, "Config Cluster"=w148, "getAll"=w156, "UI Cluster"=w150) -> (w162:T6)  [unwired: 1 in]
            n59 = call <vilib>:"Add State(s) to Queue__jki_lib_state_machine.vi"("State(s) in (\"\")"=w164) -> ("States Out"=w163:string)  [unwired: 14 in]
          }
          frame "Data: Set UI Cluster" {
            # "Do not put any code in this frame.\n(It is a separator no-op. You can make a copy of this frame to create a new Data frame)"
            n60 = call <vilib>:"Add State(s) to Queue__jki_lib_state_machine.vi"("State(s) in (\"\")"=w169) -> ("States Out"=w168:string)  [unwired: 14 in]
          }
          frame "Data: Set Config Cluster" {
            # "Do not put any code in this frame.\n(It is a separator no-op. You can make a copy of this frame to create a new Data frame)"
            n61 = Unbundle By Name(w173) -> ("UI Cluster.empty weight"=w171:dbl)
            n62 = Square(x=w171) -> (x^2=w170:dbl)
            n63 = Bundle By Name(cluster=w173, "Config Cluster.Example Setting 1"=w171, "Config Cluster.Example Setting 2"=w170) -> (w172:T6)
            n64 = call <vilib>:"Add State(s) to Queue__jki_lib_state_machine.vi"("State(s) in (\"\")"=w177) -> ("States Out"=w176:string)  [unwired: 14 in]
          }
          frame "Data: Cleanup" {
            # "Cleanup any data and references, here.\n(this is called automatically, by the Macro: Exit)"
            n65 = Unbundle By Name(w178) -> ("Core.Current VI Reference"=w182:refnum<vi>)
            n66 = Close Reference(reference=w182, error in (no error)=w181) -> (error out=w180:errorcluster)
            n67 = call <vilib>:"Add State(s) to Queue__jki_lib_state_machine.vi"("State(s) in (\"\")"=w184) -> ("States Out"=w183:string)  [unwired: 14 in]
          }
          frame "---------- UI ----------" {
            # "Do not put any code in this frame.\n(It is a separator no-op. You can make a copy of this frame to create a new UI frame)"
            n68 = call <vilib>:"Add State(s) to Queue__jki_lib_state_machine.vi"("State(s) in (\"\")"=w189) -> ("States Out"=w188:string)  [unwired: 14 in]
          }
          frame "UI: Initialize" {
            # "size window to decoration box on front panel"
            # "Initialize the User Interface, here.\n(this is called automatically, by the Macro: Init)"
            n69 = call <userlib>:"Fit VI window to Largest Dec__ogtk.vi"("error in (no error)"=w192, "border spacing (2 px)"=0) -> ("error out"=w191:errorcluster)  [unwired: 4 in, 1 out]
            n70 = disable-structure shown="Disabled" {
              frame Disabled {
                n71 = control-ref of="This VI"() -> (w198:refnum<vi>)
                n72 = property class="VI"(reference=w198) -> ("Panel"=w197:refnum<vi>)  [unwired: 1 in, 2 out]
                n73 = property class="Pnl" props=["Panel"](reference=w197) -> ()  [unwired: 1 in, 3 out]
              }
              frame Enabled {
              }
            }
            n74 = invoke on="STOP" class="Bool (strict)" method="Reinit To Default"() -> ()  [unwired: 3 in, 3 out]
            n75 = call <vilib>:"Add State(s) to Queue__jki_lib_state_machine.vi"("State(s) in (\"\")"=w196) -> ("States Out"=w195:string)  [unwired: 14 in]
          }
          frame "UI: Update FP Controls" {
            # "Do not put any code in this frame.\n(It is a separator no-op. You can make a copy of this frame to create a new UI frame)"
            n76 = Unbundle By Name(w199) -> ()  [unwired: 1 out]
            n77 = call <vilib>:"Add State(s) to Queue__jki_lib_state_machine.vi"("State(s) in (\"\")"=w203) -> ("States Out"=w202:string)  [unwired: 14 in]
          }
          frame "UI: Update FP Indicators" {
            # "do this way to have nicer UI or only display what you want"
            n78 = Unbundle By Name(w211) -> ("getAll"=w213:T4, "UI Cluster"=w210:T5)
            n79 = Unbundle By Name(w213) -> ("Net Weight(lbs)"=w206:dbl)
            "Net weight" <- w206
            n80 = Unbundle By Name(w210) -> ("empty weight"=w205:dbl, "full weight"=w209:dbl)
            n81 = Subtract(x=w209, y=w205) -> (x-y=w208:dbl)
            n82 = Subtract(x=w206, y=w205) -> (x-y=w204:dbl)
            n83 = Divide(x=w204, y=w208) -> (x/y=→"Level (%)":dbl)
            n84 = call <vilib>:"Add State(s) to Queue__jki_lib_state_machine.vi"("State(s) in (\"\")"=w216) -> ("States Out"=w215:string)  [unwired: 14 in]
          }
          frame "UI: Cursor Set" {
            # "Argument"
            # "Initialize the User Interface, here.\n(this is called automatically, by the Macro: Init)"
            n85 = disable-structure shown="Default" {
              disable-tunnel: w219 -> [w224 w227]
              disable-tunnel: [w224 w226] -> w218
              disable-tunnel: w217 -> [_ w225]
              frame condition #0 {
              }
              frame condition #1 (active) {
                n86 = case shown="\"Idle\", Default" w225 {
                  tunnel: w227 -> [w229 w231]
                  tunnel: [w228 w230] -> w226
                  frame "Idle", Default {
                    n87 = call <vilib>:"Unset Busy.vi"("error in (no error)"=w229) -> ("error out"=w228:errorcluster)  [unwired: 10 in]
                  }
                  frame "Busy" {
                    n88 = call <vilib>:"Set Busy.vi"("error in (no error)"=w231) -> ("error out"=w230:errorcluster)  [unwired: 9 in, 1 out]
                  }
                }
              }
            }
            n89 = call <vilib>:"Add State(s) to Queue__jki_lib_state_machine.vi"("State(s) in (\"\")"=w223) -> ("States Out"=w222:string)  [unwired: 14 in]
          }
          frame "UI: Front Panel State" {
            # "Argument"
            # "Set Front Panel Open or Closed\n(Usage: \"UI: Front Panel State >> Open|Close\")"
            n90 = Unbundle By Name(w235) -> ("Core.Current VI Reference"=w234:refnum<vi>)
            n91 = disable-structure shown="Default" {
              disable-tunnel: w237 -> [w243 w266]
              disable-tunnel: [w242 w266] -> w236
              disable-tunnel: w234 -> [w241 _]
              disable-tunnel: w233 -> [w240 _]
              frame condition #0 (active) {
                n92 = case shown="\"Close\"" w240 {
                  tunnel: w243 -> [w247 w260]
                  tunnel: [w249 w261] -> w242
                  tunnel: w241 -> [w248 w258]
                  frame "Open", Default {
                    n93 = property class="VI"(reference=w248, error in=w247) -> (reference out=w245:refnum<vi>, error out=w246:errorcluster, "FP.State"=w244:T2)
                    n94 = case shown="\"Closed\"" w244 {
                      tunnel: [w252 w255] -> w249
                      tunnel: w246 -> [w251 w255]
                      tunnel: w245 -> [w250 _]
                      frame "Closed" {
                        n95 = invoke class="VI" method="FP.Open"(reference=w250, error in=w251, "Activate"=TRUE, "State"=T2."Standard") -> (error out=w252:errorcluster)  [unwired: 1 in, 4 out]
                      }
                      frame Default {
                      }
                    }
                  }
                  frame "Close" {
                    n96 = property class="VI"(reference=w258, error in=w260) -> (reference out=w257:refnum<vi>, error out=w259:errorcluster, "FP.State"=w256:T2)
                    n97 = case shown="Default" w256 {
                      tunnel: [w262 w265] -> w261
                      tunnel: w259 -> [w262 w264]
                      tunnel: w257 -> [_ w263]
                      frame "Invalid", "Closed" {
                      }
                      frame Default {
                        n98 = invoke class="VI" method="FP.Close"(reference=w263, error in=w264) -> (error out=w265:errorcluster)  [unwired: 1 in, 2 out]
                      }
                    }
                  }
                }
              }
              frame condition #1 {
              }
            }
            n99 = call <vilib>:"Add State(s) to Queue__jki_lib_state_machine.vi"("State(s) in (\"\")"=w239) -> ("States Out"=w238:string)  [unwired: 14 in]
          }
          frame "---------- Macro ----------" {
            # "Do not put any code in this frame.\n(It is a separator no-op. You can make a copy of this frame to create a new Macro frame)"
            n100 = call <vilib>:"Add State(s) to Queue__jki_lib_state_machine.vi"("State(s) in (\"\")"=w271) -> ("States Out"=w270:string)  [unwired: 14 in]
          }
          frame "Macro: Initialize" {
            w274 = "UI: Initialize\nMacro: Read UI Config\n//UI: Front Panel State >> Open"  # UI: Initialize Macro: Read UI Config //UI: Front Panel State >> Open
            # "Initialization Macro\n(This is called once, when the VI starts)"
            n101 = call <vilib>:"Add State(s) to Queue__jki_lib_state_machine.vi"("State(s) in Front (\"\")"="Data: Initialize\nInitialize Core Data\nEvents: Register", "State(s) in (\"\")"="Process: Sync", "State(s) at Back (\"\")"=w274) -> ("States Out"=w273:string)  [unwired: 12 in]
            n102 = call <vilib>:"Add State(s) to Queue__jki_lib_state_machine.vi"("State(s) in Front (\"\")"=w273, "State(s) in (\"\")"=w280) -> ("States Out"=w279:string)  [unwired: 13 in]
          }
          frame "Macro: Read UI Config" {
            # "Do not put any code in this frame.\n(It is a separator no-op. You can make a copy of this frame to create a new Macro frame)"
            n103 = call <vilib>:"Add State(s) to Queue__jki_lib_state_machine.vi"("State(s) in Front (\"\")"="Configuration: Initialize\nConfiguration: Read UI Config File\nUI: Update FP Controls" ("State(s) in Front (\"\")"), "State(s) in (\"\")"=w286) -> ("States Out"=w285:string)  [unwired: 13 in]
          }
          frame "Macro: Write UI Config" {
            # "Do not put any code in this frame.\n(It is a separator no-op. You can make a copy of this frame to create a new Macro frame)"
            n104 = call <vilib>:"Add State(s) to Queue__jki_lib_state_machine.vi"("State(s) in Front (\"\")"="Data: Set UI Cluster\nConfiguration: Write UI Config File" ("State(s) in Front (\"\")"), "State(s) in (\"\")"=w292) -> ("States Out"=w291:string)  [unwired: 13 in]
          }
          frame "Macro: Exit" {
            # "Exit Macro\n(This is called once, when the VI exits)"
            n105 = Unbundle By Name(w294) -> ("Core.Close Panel on Exit?"=w304:bool)
            n106 = Select(t="UI: Front Panel State >> Close", s=w304, f="") -> (s? t:f=w301:string)
            n107 = call <vilib>:"Add State(s) to Queue__jki_lib_state_machine.vi"("State(s) in Front (\"\")"="Data: Cleanup\nEvents: Unregister\nProcess: Self Terminate", "State(s) in (\"\")"="Process: Sync", "State(s) at Back (\"\")"="Exit") -> ("States Out"=w296:string)  [unwired: 12 in]
            n108 = call <vilib>:"Add State(s) to Queue__jki_lib_state_machine.vi"("State(s) in Front (\"\")"="Macro: Write UI Config", "State(s) in (\"\")"=w301, "State(s) at Back (\"\")"=w296) -> ("States Out"=w300:string)  [unwired: 12 in]
            n109 = call <vilib>:"Add State(s) to Queue__jki_lib_state_machine.vi"("State(s) in Front (\"\")"=w300, "State(s) in (\"\")"=w307) -> ("States Out"=w306:string)  [unwired: 13 in]
          }
          frame "---------- Process ----------" {
            # "Template Separator\n(You can make a copy of, or modify, this frame)"
            n110 = call <vilib>:"Add State(s) to Queue__jki_lib_state_machine.vi"("State(s) in (\"\")"=w312) -> ("States Out"=w311:string)  [unwired: 14 in]
          }
          frame "Process: Sync" {
            n111 = Unbundle By Name(w320) -> ("Instrument UI"=w316:refnum<class "Instrument UI.LN2.lvclass">)
            n112 = call <vilib>:"WaitOnProcessSync.vi"("error in (no error)"=w315, "SMO"=w316) -> ("error out"=w314:errorcluster, "Don't run?"=w319:bool)  [unwired: 7 in, 1 out]
            n113 = Select(t="Data: Cleanup\nEvents: Unregister\nExit", s=w319, f="") -> (s? t:f=w313:string)
            n114 = call <vilib>:"Add State(s) to Queue__jki_lib_state_machine.vi"("State(s) in Front (\"\")"=w313, "State(s) in (\"\")"=w323) -> ("States Out"=w322:string)  [unwired: 13 in]
          }
          frame "Process: Self Terminate" {
            n115 = Unbundle By Name(w325) -> ("Instrument UI"=w324:refnum<class "Instrument UI.LN2.lvclass">)
            n116 = call <vilib>:"SelfTerminate.vi"("error in (no error)"=w327, "SMO in"=w324) -> ("error out"=w326:errorcluster)  [unwired: 8 in, 1 out]
            n117 = call <vilib>:"Add State(s) to Queue__jki_lib_state_machine.vi"("State(s) in (\"\")"=w330) -> ("States Out"=w329:string)  [unwired: 14 in]
          }
          frame "---------- Events ----------" {
            # "Template Separator\n(You can make a copy of, or modify, this frame)"
            n118 = call <vilib>:"Add State(s) to Queue__jki_lib_state_machine.vi"("State(s) in (\"\")"=w335) -> ("States Out"=w334:string)  [unwired: 14 in]
          }
          frame "Events: Register" {
            # "Expand to add\nmore events"
            # "Base Class Protected Events"
            n119 = Unbundle By Name(w346) -> ("Instrument UI"=w337:refnum<class "Instrument UI.LN2.lvclass">, "Instrument"=w336:refnum<class "Instrument.LN2.lvclass">)
            n120 = call <vilib>:"GetProtectedEvents.vi"("SMO"=w337) -> ("error out"=w340:errorcluster, "SMO Protected Events"=w344:T8)  [unwired: 8 in, 1 out]
            n121 = call <userlib>:"Instrument.GetPublicEvents.vi"("Instrument"=w336) -> ("error out"=w338:errorcluster, "Instrument Public Events"=w339:T9)  [unwired: 8 in, 1 out]
            n122 = register-events(w344, w339) -> (reference out=w345:refnum<event-registration>, error out=w342:errorcluster)  [unwired: 2 in]
            n123 = Merge Errors(w338, w343, w342, w340) -> (w341:errorcluster)
            n124 = call <vilib>:"Add State(s) to Queue__jki_lib_state_machine.vi"("State(s) in (\"\")"=w348) -> ("States Out"=w347:string)  [unwired: 14 in]
          }
          frame "Events: Unregister" {
            n125 = Unregister For Events(event registration refnum=w351, error in=w350) -> (error out=w349:errorcluster)
            n126 = call <vilib>:"Add State(s) to Queue__jki_lib_state_machine.vi"("State(s) in (\"\")"=w354) -> ("States Out"=w353:string)  [unwired: 14 in]
          }
          frame "---------- Configuration ----------" {
            # "Do not put any code in this frame.\n(It is a separator no-op. You can make a copy of this frame to create a new UI frame)"
            n127 = call <vilib>:"Add State(s) to Queue__jki_lib_state_machine.vi"("State(s) in (\"\")"=w359) -> ("States Out"=w358:string)  [unwired: 14 in]
          }
          frame "Configuration: Initialize" {
            # "Do not put any code in this frame.\n(It is a separator no-op. You can make a copy of this frame to create a new UI frame)"
            n128 = Unbundle By Name(w367) -> ("Configuration"=w365:refnum<class "Configuration.lvclass">, "Instrument"=w366:refnum<class "Instrument.LN2.lvclass">)
            n129 = call <vilib>:"GetName.vi"("error in (no error)"=w369, "SMO"=w366) -> ("error out"=w368:errorcluster, "Name"=w370:string)  [unwired: 6 in, 2 out]
            n130 = call <userlib>:"Default Path.vi"("error in (no error)"=w368, "Folder Name [Application Name]"=w370, "Configuration in"=w365) -> ("error out"=w362:errorcluster, "Configuration out"=w364:refnum<class "Configuration.lvclass">)  [unwired: 7 in]
            n131 = call <userlib>:"Write Section.vi"("error in (no error)"=w362, "Section"="UI", "Configuration in"=w364) -> ("error out"=w361:errorcluster, "Configuration out"=w363:refnum<class "Configuration.lvclass">)  [unwired: 7 in]
            n132 = Bundle By Name(cluster=w367, "Configuration"=w363) -> (w371:T6)
            n133 = call <vilib>:"Add State(s) to Queue__jki_lib_state_machine.vi"("State(s) in (\"\")"=w374) -> ("States Out"=w373:string)  [unwired: 14 in]
          }
          frame "Configuration: Write UI Config File" {
            # "Do not put any code in this frame.\n(It is a separator no-op. You can make a copy of this frame to create a new Data frame)"
            n134 = Unbundle By Name(w379) -> ("Configuration"=w376:refnum<class "Configuration.lvclass">, "UI Cluster"=w378:T5)
            n135 = call <userlib>:"Write Configuration.vi"("error in (no error)"=w375, "Variant"=w378, "Configuration in"=w376) -> ("error out"=w377:errorcluster)  [unwired: 7 in, 1 out]
            n136 = call <vilib>:"Add State(s) to Queue__jki_lib_state_machine.vi"("State(s) in (\"\")"=w382) -> ("States Out"=w381:string)  [unwired: 14 in]
          }
          frame "Configuration: Read UI Config File" {
            # "Do not put any code in this frame.\n(It is a separator no-op. You can make a copy of this frame to create a new UI frame)"
            n137 = Unbundle By Name(w385) -> ("UI Cluster"=w388:T5, "Configuration"=w391:refnum<class "Configuration.lvclass">)
            n138 = call <userlib>:"Read Configuration.vi"("INI Fomatted Cluster Type"=w388, "error in (no error)"=w387, "Configuration in"=w391) -> ("error out"=w390:errorcluster, "Configuration"=w389:variant)  [unwired: 6 in, 1 out]
            n139 = Variant To Data(error in=w390, type=w388, Variant=w389) -> (data=w384:T5, error out=w386:errorcluster)
            n140 = Bundle By Name(cluster=w385, "UI Cluster"=w384) -> (w383:T6)
            n141 = call <vilib>:"Add State(s) to Queue__jki_lib_state_machine.vi"("State(s) in (\"\")"=w394) -> ("States Out"=w393:string)  [unwired: 14 in]
          }
          frame "---------- Action ----------" {
            n142 = Unbundle By Name(w397) -> ("Instrument UI"=w395:refnum<class "Instrument UI.LN2.lvclass">)
            n143 = Bundle By Name(cluster=w397, "Instrument UI"=w395) -> (w396:T6)
            n144 = call <vilib>:"Add State(s) to Queue__jki_lib_state_machine.vi"("State(s) in (\"\")"=w401) -> ("States Out"=w400:string)  [unwired: 14 in]
          }
          frame "Action: Notify UI Closed" {
            # "Notify that the UI has been closed"
            n145 = Unbundle By Name(w402) -> ("Instrument UI"=w405:refnum<class "Instrument UI.LN2.lvclass">)
            n146 = call <vilib>:"Hide.vi"("error in (no error)"=w404, "SMO.UI"=w405) -> ("error out"=w403:errorcluster)  [unwired: 8 in, 1 out]
            n147 = call <vilib>:"Add State(s) to Queue__jki_lib_state_machine.vi"("State(s) in (\"\")"=w408) -> ("States Out"=w407:string)  [unwired: 14 in]
          }
          frame "Action: getAll" {
            n148 = Unbundle By Name(w415) -> ("getAll"=w409:T4, "Instrument"=w414:refnum<class "Instrument.LN2.lvclass">)
            n149 = call "GET ALL.vim"("type"=w409, "error in (no error)"=w411, "Instrument in"=w414) -> ("error out"=w410:errorcluster, "getAll"=w412:T4, "Instrument out"=w413:refnum<class "Instrument.LN2.lvclass">)  [unwired: 6 in]
            n150 = Bundle By Name(cluster=w415, "Instrument"=w413, "getAll"=w412) -> (w416:T6)
            n151 = call <vilib>:"Add State(s) to Queue__jki_lib_state_machine.vi"("State(s) in Front (\"\")"="" ("State(s) in Front (\"\")"), "State(s) in (\"\")"=w420) -> ("States Out"=w419:string)  [unwired: 13 in]
          }
          frame "Action: setConfiguration" {
            n152 = Unbundle By Name(w423) -> ("Instrument"=w426:refnum<class "Instrument.LN2.lvclass">, "Config Cluster"=w421:T3)
            n153 = call "SET CONFIG.vim"("error in (no error)"=w424, "Configuration"=w421, "Instrument in"=w426) -> ("error out"=w428:errorcluster, "Instrument out"=w422:refnum<class "Instrument.LN2.lvclass">)  [unwired: 7 in]
            n154 = Bundle By Name(cluster=w423, "Instrument"=w422) -> (w425:T6)
            n155 = call <vilib>:"Add State(s) to Queue__jki_lib_state_machine.vi"("State(s) in Front (\"\")"="" ("State(s) in Front (\"\")"), "State(s) in (\"\")"=w431) -> ("States Out"=w430:string)  [unwired: 13 in]
          }
          frame "Action: Sayanwita 1" {
            n156 = Unbundle By Name(w436) -> ("Instrument"=w434:refnum<class "Instrument.LN2.lvclass">)
            n157 = call "Remote Client.vim"("method"="awesome_command_1", "Instrument in"=w434) -> ("Instrument out"=w433:refnum<class "Instrument.LN2.lvclass">)  [unwired: 6 in, 3 out]
            n158 = Bundle By Name(cluster=w436, "Instrument"=w433) -> (w435:T6)
            n159 = call <vilib>:"Add State(s) to Queue__jki_lib_state_machine.vi"("State(s) in (\"\")"=w440) -> ("States Out"=w439:string)  [unwired: 14 in]
          }
          frame "Action: Sayanwita 1 (copy)" {
            n160 = Unbundle By Name(w445) -> ("Instrument"=w443:refnum<class "Instrument.LN2.lvclass">)
            n161 = call <userlib>:"Instrument.MessageToProcess.vi"("Command"="awesome_command_2", "Instrument"=w443) -> ("Instrument out"=w441:refnum<class "Instrument.LN2.lvclass">)  [unwired: 8 in, 1 out]
            n162 = Bundle By Name(cluster=w445, "Instrument"=w441) -> (w444:T6)
            n163 = call <vilib>:"Add State(s) to Queue__jki_lib_state_machine.vi"("State(s) in (\"\")"=w449) -> ("States Out"=w448:string)  [unwired: 14 in]
          }
        }
      }
    }
    frame Error {
    }
  }
  n164 = call-parent "Process.vi"("error in"=w5, "Instrument UI in"=w4) -> ("error out"=w2:errorcluster, "Instrument UI out"=→"Example Instrument UI out":refnum<class "Instrument UI.LN2.lvclass">)  [unwired: 8 in]
  n165 = Merge Errors(w2, w1) -> (→"error out":errorcluster)
